vi "WT500 Read Power.vi"(0 "VISA resource name":refnum<visa-resource-name>="WT500", 1 "WT500 CMDS":T1, 5 "V Range (8: 1000V)":u16(ring)=6 items=["AUTO", "15", "30", "60", "100", "150", "300", "600", "1000", "7.5", "15", "30", "50", "75", "150", "300", "500"], 7 "I Range (7: 40A)":u16(ring)=7 items=["AUTO", "500 mA", "1 A", "2 A", "5 A", "10 A", "20 A", "40 A", "S-AUTO", "50 mV", "100 mV", "200 mV", "500 mV", "1 V", "2 V", "5 V", "10 V", "250 mA", "500 mA", "1 A", "2.5 A", "5 A", "10 A", "20 A", "25 mV", "50 mV", "100 mV", "250 mV", "500 mV", "1 V", "2.5 V", "5 V"], 11 "error in (no error)":errorcluster) -> (4 "VISA resource name out":refnum<visa-resource-name>="WT500", 6 "PowerData":T2={"Current L1"=236.2, "Current L2"=17.749, "Power"=4192.0, "WattHours"=0.0, "Voltage L2"=236.2, "Voltage L1"=236.2}, 8 "Error Message":string, 10 "Measurement Values":dbl[](array[numeric]) format="%.4p", 14 "Label":string[](array[string])=["Urms:Element 1", "Urms:Element 2", "Irms:Element 1", "Irms:Element 2", "P:Sigma", "Wp:Sigma", "I +peak:Element 1", "I +peak:Element 2"], 15 "error out":errorcluster)   [LabVIEW 2012]
uses:
  Dryer PowerData.ctl
  WT500 Sequences.ctl
  Drivers/Yokogawa WT200 Series/Yokogawa WT200 Series.lvlib
panel:
  out "Error Message 2":string
  out "(Max Current)":dbl
  in  "Pole":u16(ring)=1 items=["NONE", "Element 1", "Element 2", "Element 3", "Sigma"]
  in  "Measurement":u16(ring)=1 items=["None", "Urms", "Umn", "Udc", "Urmn", "Uac", "Irms", "Imn", "Idc", "Irmn", "Iac", "P", "S", "Q", "Lambda", "Phi", "Freq U", "Freq I", "U +peak", "U -peak", "I +peak", "I -peak", "Cf U", "Cf I", "Time", "Wp", "Wp+", "Wp-", "q", "q+", "q-", "WS", "WQ", "Eta 1", "Eta 2", "F1", "F2", "F3", "F4", "F5", "F6", "F7", "F8", "U(k)", "I(k)", "P(k)", "S(k)", "Q(k)", "Lambda(k)", "Phi(k)", "Phi U(k)", "Phi I(k)", "Uhdf(k)", "Ihdf(k)", "Phdf(k)", "Uthd", "Ithd", "Pthd", "Phi Ui-Uj", "Phi Ui-Uk", "Phi Ui-Ii", "Phi Ui-Ij", "Phi Ui-Ik", "Delta 1", "Delta 2", "Delta 3", "Delta 4"]
  out "Data Length":i32
  out "Read Data":string
  in  "Write Data":string
  out "Scan Error":bool
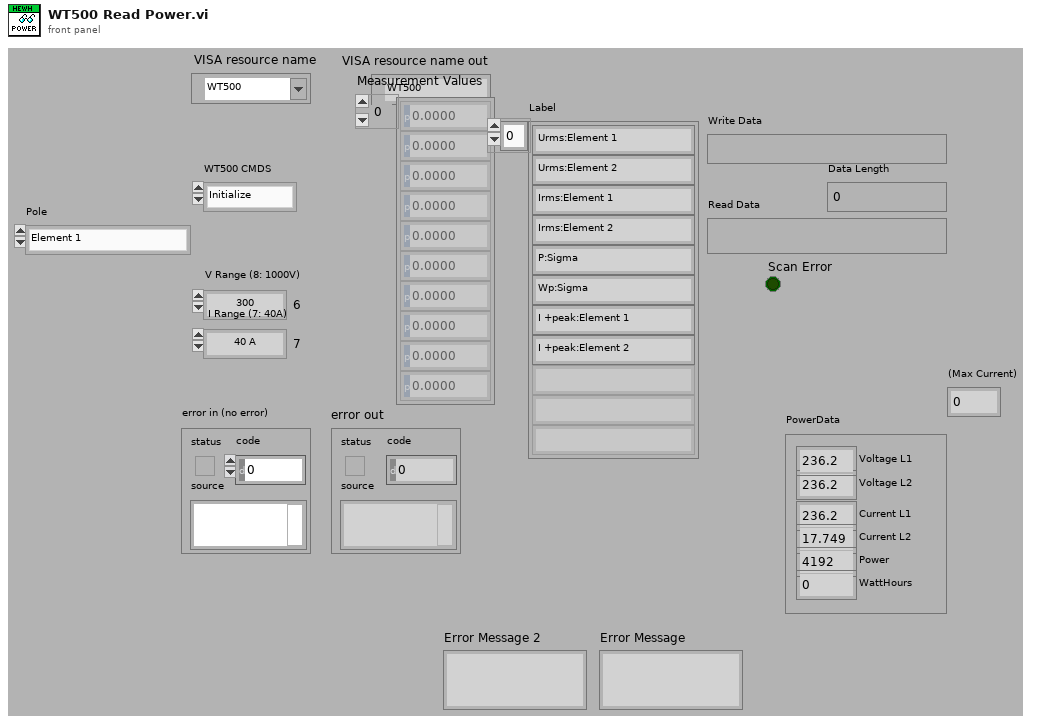
[diagram p1: front panel]
types:
  T1 = typedef "WT500 Sequences.ctl" = enum16{"Initialize", "GetReadings", "GetErrors", "Close", "NoOp", "MiscCmd"}
  T2 = typedef "Dryer PowerData.ctl" = cluster{"Current L1":dbl, "Current L2":dbl, "Power":dbl, "WattHours":dbl, "Voltage L2":dbl, "Voltage L1":dbl}
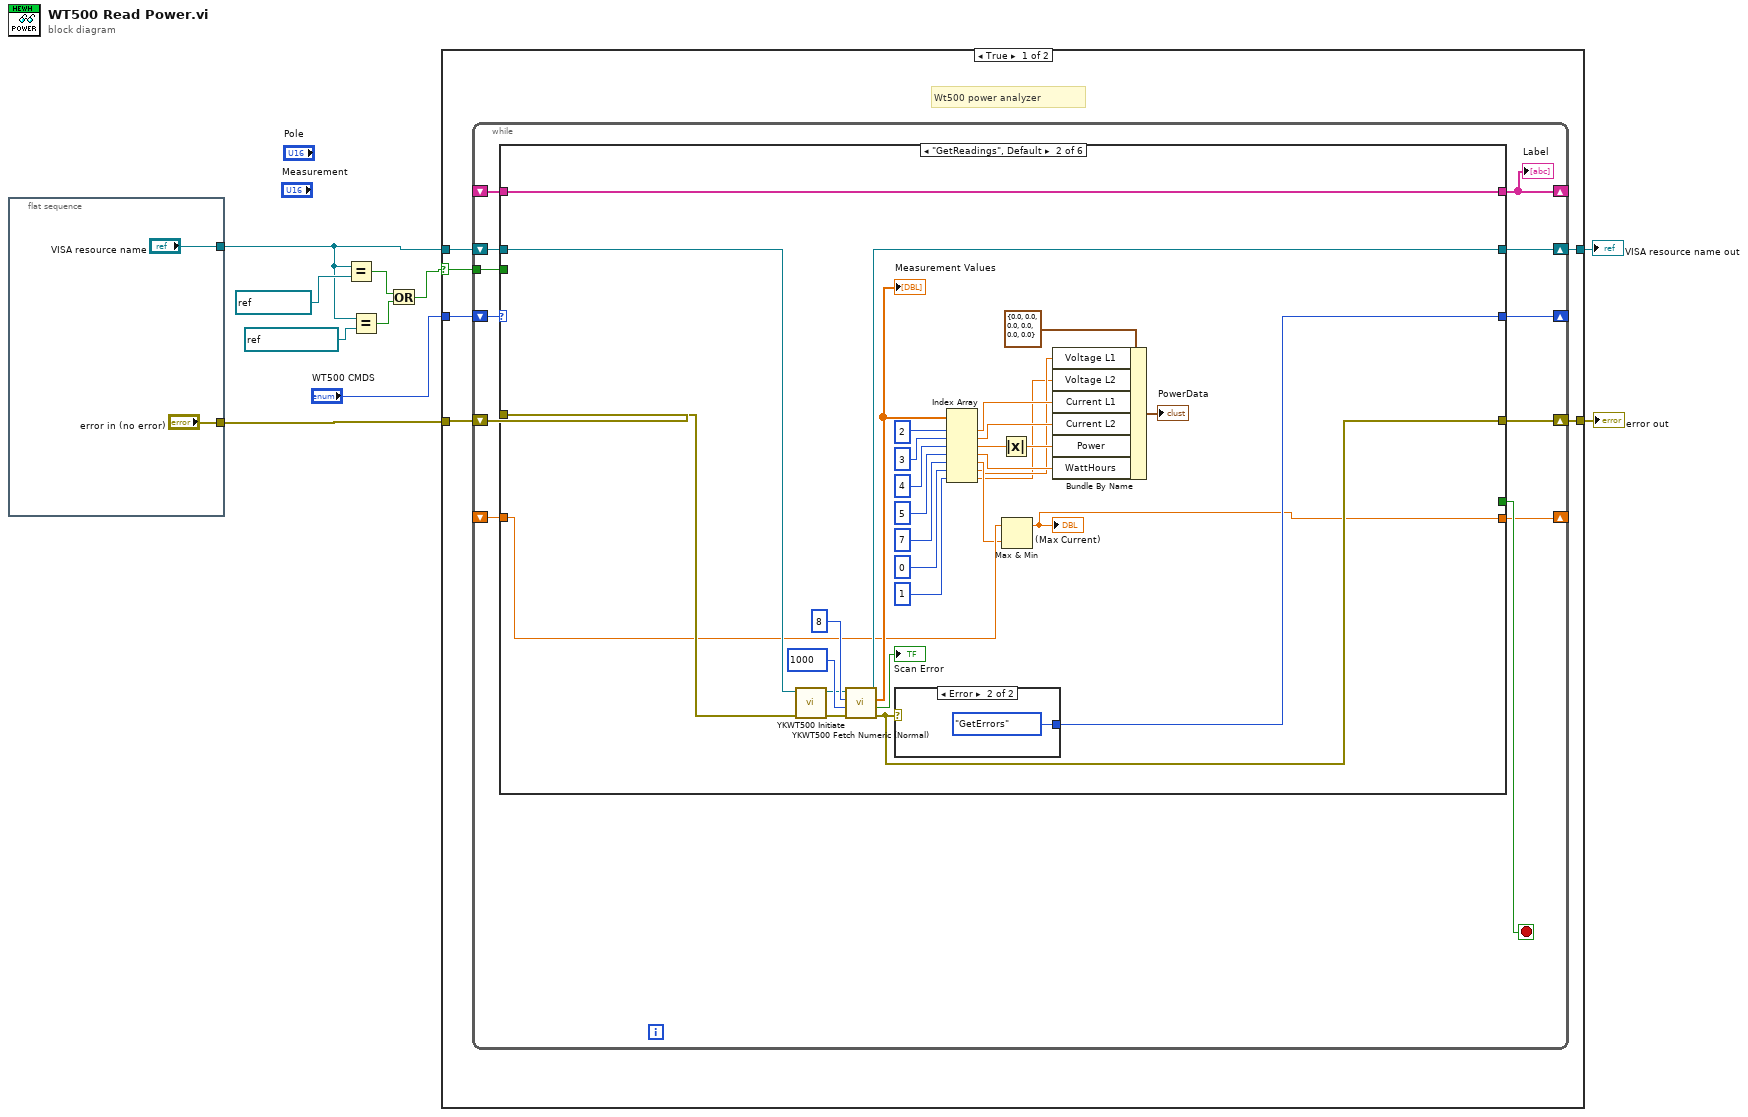
[diagram p0: block diagram]
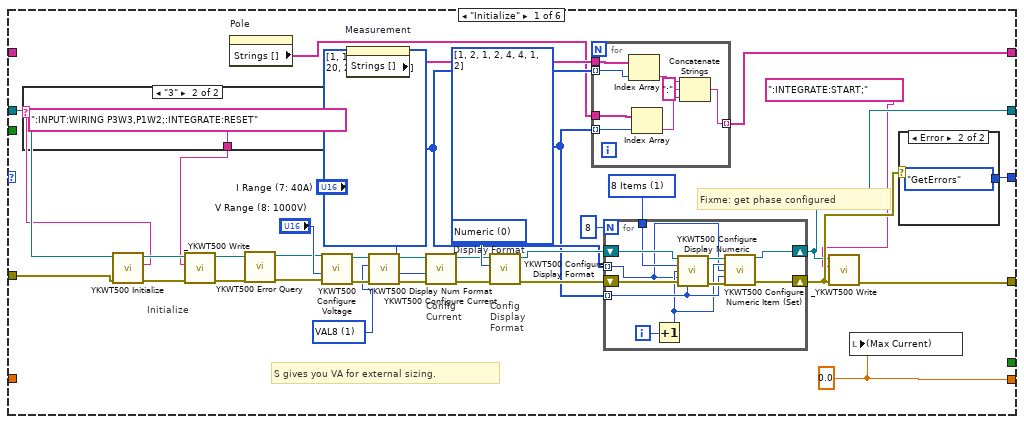
[diagram p2: hidden frame]
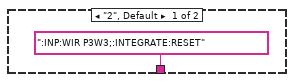
[diagram p3: hidden frame]
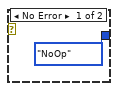
[diagram p4: hidden frame]
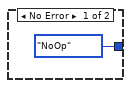
[diagram p5: hidden frame]
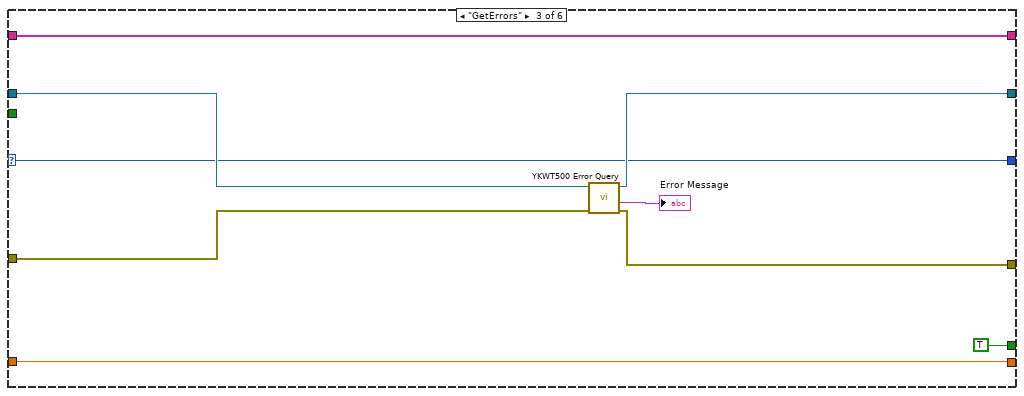
[diagram p6: hidden frame]
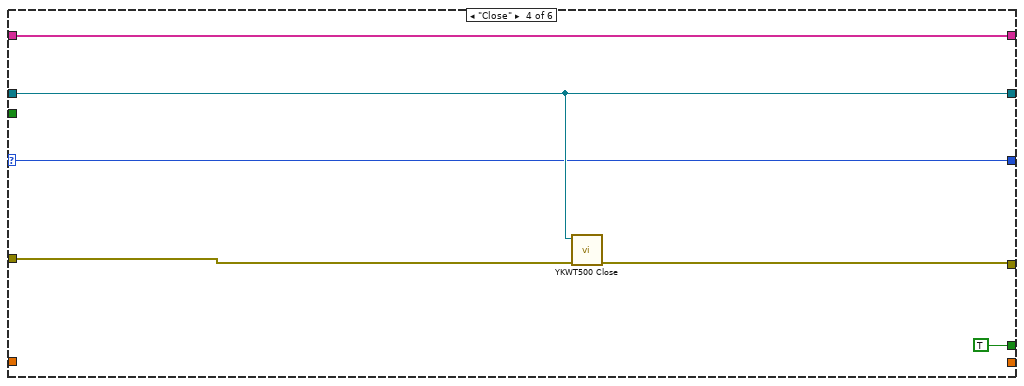
[diagram p7: hidden frame]
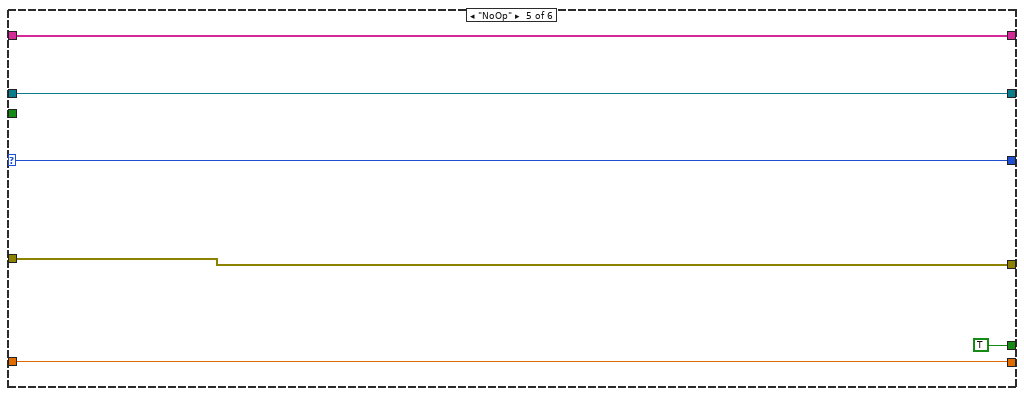
[diagram p8: hidden frame]
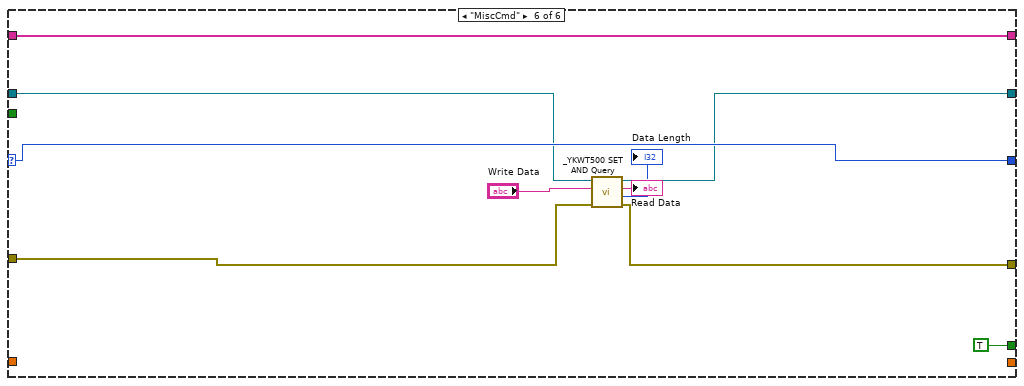
[diagram p9: hidden frame]
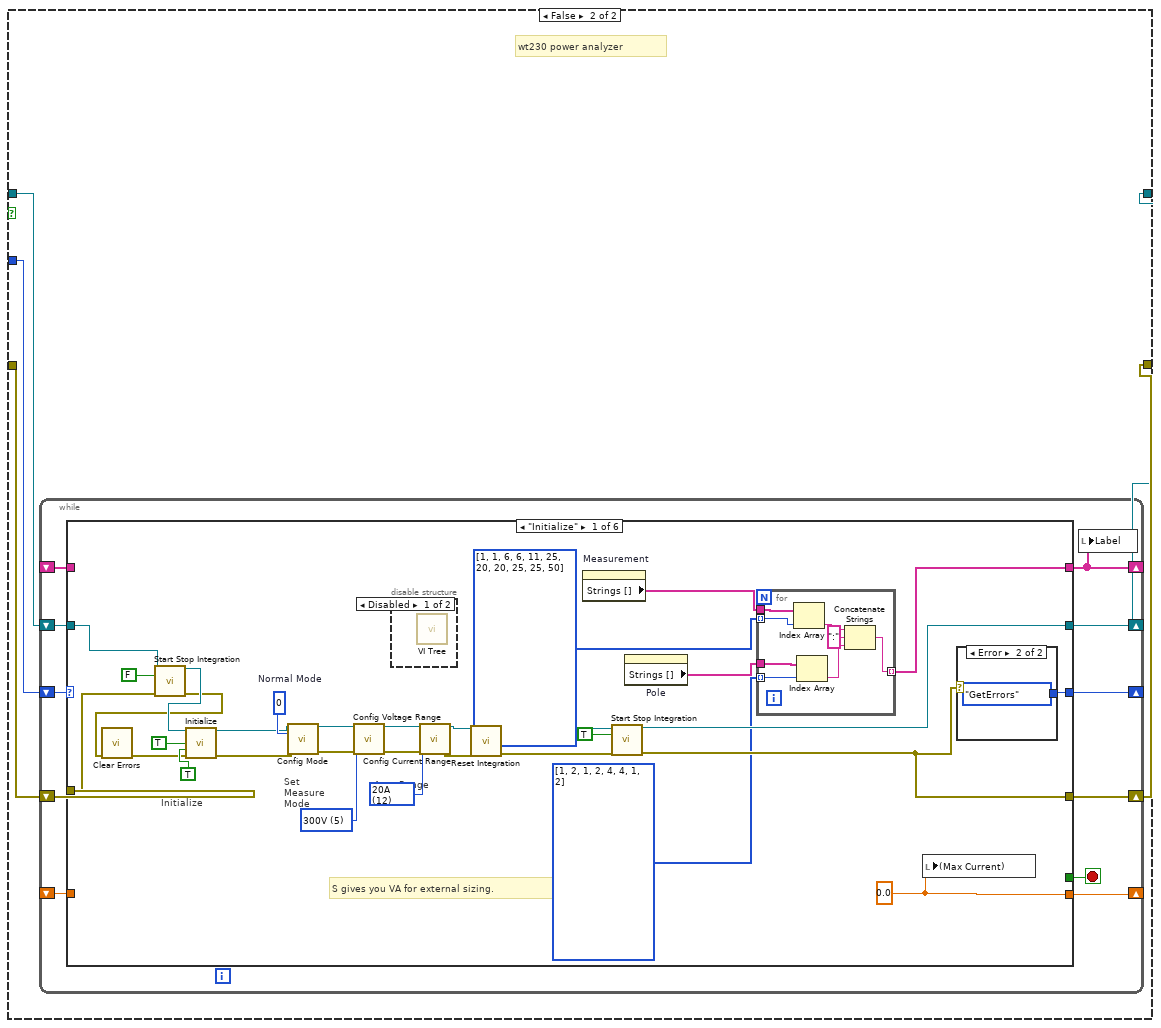
[diagram p10: hidden frame]
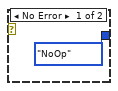
[diagram p12: hidden frame]
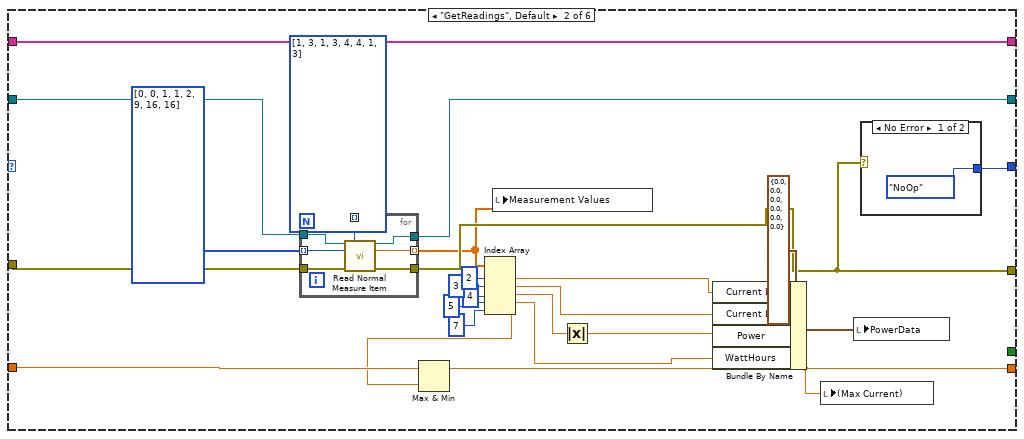
[diagram p13: hidden frame]
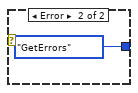
[diagram p14: hidden frame]
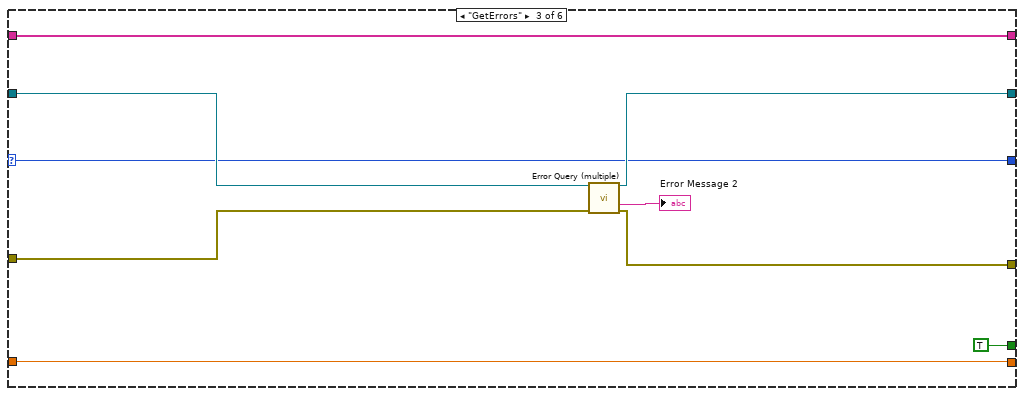
[diagram p15: hidden frame]
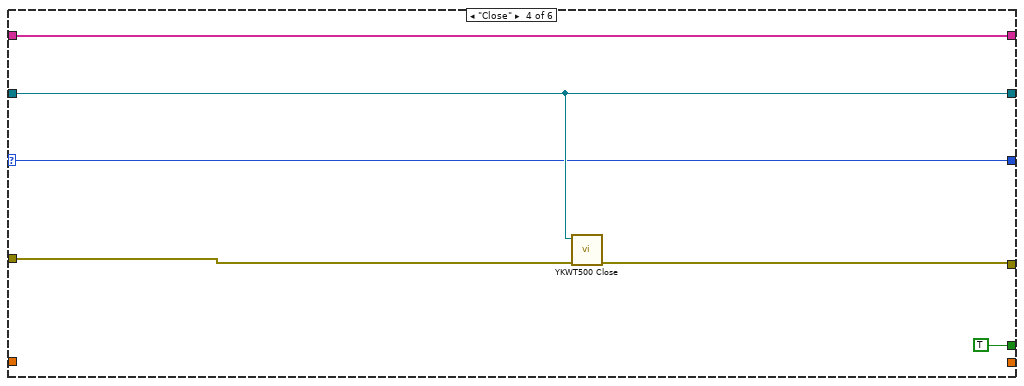
[diagram p16: hidden frame]
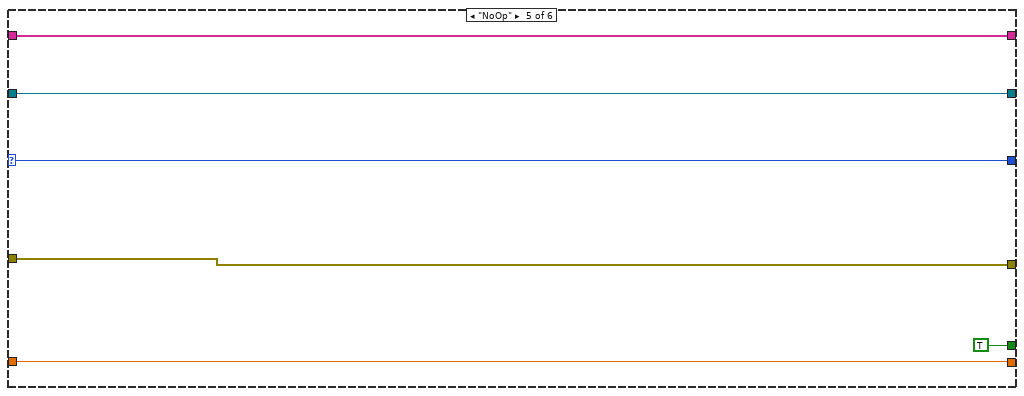
[diagram p17: hidden frame]
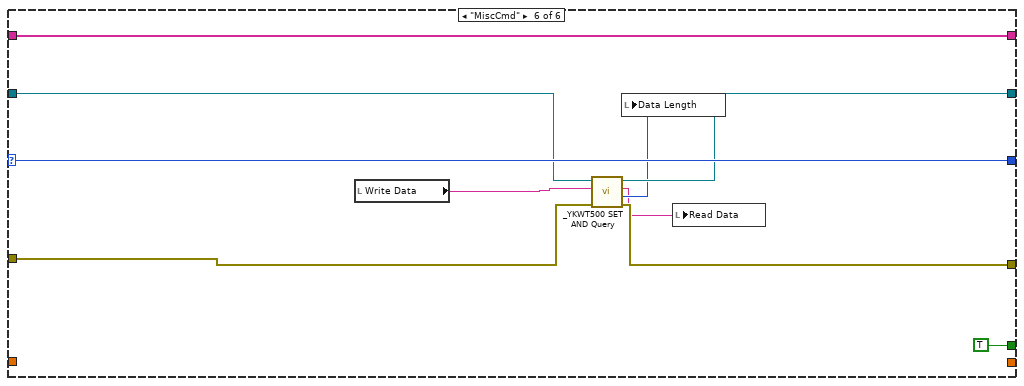
[diagram p18: hidden frame]
diagram:
  n1 = flat-sequence {
    tunnel: ["error in (no error)"] -> w7
    tunnel: ["VISA resource name"] -> w5
    frame #0 {
    }
  }
  n2 = Equal?(x=w5, y=refnum<visa-resource-name> "WT500" ("VISA resource name")) -> (x = y?=w2:bool)
  n3 = Equal?(x=w5, y=refnum<visa-resource-name> "YGWT500" ("VISA resource name")) -> (x = y?=w3:bool)
  n4 = Or(x=w2, y=w3) -> (x .or. y?=w1:bool)
  n5 = case shown="True" w1 {
    selector: w1 -> [w13 _]
    tunnel: "WT500 CMDS" -> [w18 w157]
    tunnel: w7 -> [w17 w156]
    tunnel: [w16 w155] -> w9
    tunnel: w5 -> [w15 w154]
    tunnel: [w14 w153] -> w8
    frame True {
      # "Wt500 power analyzer"
      n6 = while {
        shift-right: [w28] -> w16
        shift-left: w17 -> [w29]
        shift-right: [w26] -> _
        shift-left: w18 -> [w30]
        shift-right: [w24] -> w14
        shift-left: w15 -> [w25]
        shift-right: [w22] -> _
        shift-left: _ -> [w23]
        shift-right: [w21] -> _
        shift-left: _ -> [w20]
        tunnel: w13 -> [w19]
        stop <- w27 stop-if-true
        n7 = case shown="\"GetReadings\", Default" w30 {
          selector: w30 -> [_ _ w126 w133 w140 w151]
          tunnel: w29 -> [w60 w100 w128 w136 w141 w148]
          tunnel: [w37 w103 w124 w135 w141 w147] -> w28
          tunnel: [_ _ TRUE TRUE TRUE TRUE] -> w27
          tunnel: [w59 w102 w126 w133 w140 w151] -> w26
          tunnel: w25 -> [w58 w101 w130 w134 w139 w150]
          tunnel: [w38 w104 w129 w134 w139 w149] -> w24
          tunnel: [w44 w97 w123 w131 w138 w143] -> w22
          tunnel: w23 -> [_ w97 w123 w131 w138 w143]
          tunnel: [w40 w93 w122 _ w137 _] -> w21
          tunnel: w20 -> [_ w95 w122 _ w137 _]
          tunnel: w19 -> [_ _ _ _ _ _]
          frame "Initialize" {
            w40 = 0.0
            w49 = u16 1 items=["VAL4", "VAL8", "VAL16", "MATRIX", "ALL"] ("Display Format (0: Numeric)")
            w46 = u16[] [1, 2, 1, 2, 4, 4, 1, 2] items=["NONE", "Element 1", "Element 2", "Element 3", "Sigma"]
            w48 = u16[] [1, 1, 6, 6, 11, 25, 20, 20, 25, 25, 50] items=["None", "Urms", "Umn", "Udc", "Urmn", "Uac", "Irms", "Imn", "Idc", "Irmn", "Iac", "P", "S", "Q", "Lambda", "Phi", "Freq U", "Freq I", "U +peak", "U -peak", "I +peak", "I -peak", "Cf U", "Cf I", "Time", "Wp", "Wp+", "Wp-", "q", "q+", "q-", "WS", "WQ", "Eta 1", "Eta 2", "F1", "F2", "F3", "F4", "F5", "F6", "F7", "F8", "U(k)", "I(k)", "P(k)", "S(k)", "Q(k)", "Lambda(k)", "Phi(k)", "Phi U(k)", "Phi I(k)", "Uhdf(k)", "Ihdf(k)", "Phdf(k)", "Uthd", "Ithd", "Pthd", "Phi Ui-Uj", "Phi Ui-Uk", "Phi Ui-Ii", "Phi Ui-Ij", "Phi Ui-Ik", "Delta 1", "Delta 2", "Delta 3", "Delta 4"] ("Array of Measurements")
            w55 = u16 1 items=["4 Items", "8 Items", "16 Items", "Matrix"] ("Numeric Format (0: 4 Items)")
            w65 = u16 0 items=["Numeric", "Wave", "Bar", "Vector", "Trend"]  # Display Format
            # "S gives you VA for external sizing."
            # "Fixme: get phase configured"
            # "Config\nDisplay\nFormat"
            # "Config\nCurrent"
            # "Config\nVoltage"
            # "Initialize"
            n8 = call "YKWT500 Initialize.vi"("error in (no error)"=w60, "VISA resource name"=w58) -> ("error out"=w42:errorcluster, "Num Cards"=w31:string, "VISA resource name out"=w43:refnum<visa-resource-name>)  [unwired: 7 in]
            n9 = case shown="\"3\"" w31 {
              tunnel: [":INP:WIR P3W3;:INTEGRATE:RESET" ("Write Data") ":INPUT:WIRING P3W3,P1W2;:INTEGRATE:RESET" ("Write Data")] -> w41
              frame "2", Default {
              }
              frame "3" {
              }
            }
            n10 = call "_YKWT500 Write.vi"("error in (no error)"=w42, "Write Data"=w41, "VISA resource name"=w43) -> ("error out"=w35:errorcluster, "VISA resource name out"=w34:refnum<visa-resource-name>)  [unwired: 5 in, 2 out]
            n11 = property on="Pole" class="Ring (strict)"() -> ("Strings []"=w45:string[])  [unwired: 2 in, 2 out]
            n12 = call "YKWT500 Error Query.vi"("error in (no error)"=w35, "VISA resource name"=w34) -> ("error out"=w32:errorcluster, "VISA resource name out"=w33:refnum<visa-resource-name>)  [unwired: 6 in, 2 out]
            n13 = call "YKWT500 Configure Voltage.vi"("error in (no error)"=w32, "Voltage Range (8: 1000V)"="V Range (8: 1000V)", "VISA resource name"=w33) -> ("error out"=w53:errorcluster, "VISA resource name out"=w50:refnum<visa-resource-name>)  [unwired: 7 in]
            n14 = property on="Measurement" class="Ring (strict)"() -> ("Strings []"=w47:string[])  [unwired: 2 in, 2 out]
            n15 = call "YKWT500 Display Num Format.vi"("error in (no error)"=w53, "Display Format (0: Numeric)"=w49, "VISA resource name"=w50) -> ("error out"=w52:errorcluster, "VISA resource name out"=w51:refnum<visa-resource-name>)  [unwired: 7 in]
            n16 = call "YKWT500 Configure Current.vi"("error in (no error)"=w52, "Current Range (7: 40A)"="I Range (7: 40A)", "VISA resource name"=w51) -> ("error out"=w64:errorcluster, "VISA resource name out"=w63:refnum<visa-resource-name>)  [unwired: 7 in]
            n17 = call "YKWT500 Configure Display Format.vi"("error in (no error)"=w64, "Display Format (0: Numeric)"=w65, "VISA resource name"=w63) -> ("error out"=w56:errorcluster, "VISA resource name out"=w57:refnum<visa-resource-name>)  [unwired: 7 in]
            n18 = for {
              tunnel: w48 -> [w75] mode=indexing
              tunnel: w47 -> [w74]
              tunnel: w46 -> [w73] mode=indexing
              tunnel: w45 -> [w72]
              tunnel: [w68] -> w44 mode=indexing
              n19 = Index Array(array=w74, index=w75) -> (element=w71:string)
              n20 = Index Array(array=w72, index=w73) -> (element=w69:string)
              n21 = Concatenate Strings(w71, ":" ("string"), w69) -> (w68:string)
            }
            n22 = for {
              N: 8 -> [_]
              shift-right: [w80] -> w38
              shift-left: w57 -> [w86]
              shift-right: [w81] -> w39
              shift-left: w56 -> [w85]
              tunnel: w55 -> [w83]
              tunnel: w46 -> [w78] mode=indexing
              tunnel: w48 -> [w76] mode=indexing
              i -> [w84]
              n23 = Increment(x=w84) -> (x+1=w77:i32)
              n24 = call "YKWT500 Configure Display Numeric.vi"("VISA resource name"=w86, "Numeric Format (0: 4 Items)"=w83, "Numeric Item Number (1)"=w77, "Numeric Function (0: None)"=w76, "error in (no error)"=w85, "Element (1: Element 1)"=w78) -> ("VISA resource name out"=w79:refnum<visa-resource-name>, "error out"=w82:errorcluster)  [unwired: 8 in]
              n25 = call "YKWT500 Configure Numeric Item (Set).vi"("VISA resource name"=w79, "Numeric Item Number (1)"=w77, "Numeric Function (0: None)"=w76, "Element (1: Element 1)"=w78, "error in (no error)"=w82) -> ("VISA resource name out"=w80:refnum<visa-resource-name>, "error out"=w81:errorcluster)  [unwired: 9 in]
            }
            n26 = call "_YKWT500 Write.vi"("error in (no error)"=w39, "Write Data"=":INTEGRATE:START;", "VISA resource name"=w38) -> ("error out"=w37:errorcluster)  [unwired: 5 in, 3 out]
            n27 = local write "(Max Current)"(w40) -> ()
            n28 = case shown="Error" w39 {
              tunnel: [WT500_Sequences."NoOp" ("WT500 CMDS") WT500_Sequences."GetErrors" ("WT500 CMDS")] -> w59
              frame No Error {
              }
              frame Error {
              }
            }
          }
          frame "GetReadings", Default {
            n29 = call "YKWT500 Initiate.vi"("error in (no error)"=w100, "VISA resource name"=w101) -> ("error out"=w98:errorcluster, "VISA resource name out"=w99:refnum<visa-resource-name>)  [unwired: 8 in]
            n30 = call "YKWT500 Fetch Numeric (Normal).vi"("error in (no error)"=w98, "Timeout (10000 ms)"=u32 1000, "Number of Item (255)"=8, "VISA resource name"=w99) -> ("error out"=w103:errorcluster, "Scan Error"=→"Scan Error":bool, "Measurement Value"=w108:dbl[], "VISA resource name out"=w104:refnum<visa-resource-name>)  [unwired: 4 in]
            "Measurement Values" <- w108
            n31 = case shown="Error" w103 {
              tunnel: [WT500_Sequences."NoOp" ("WT500 CMDS") WT500_Sequences."GetErrors" ("WT500 CMDS")] -> w102
              frame No Error {
              }
              frame Error {
              }
            }
            n32 = Index Array(array=w108, index #1=2 ("index"), index #2=3 ("index"), index #3=4 ("index"), index #4=5 ("index"), index #5=7 ("index"), index #6=0 ("index"), index #7=1 ("index")) -> (element #1=w118:dbl, element #2=w117:dbl, element #3=w112:dbl, element #4=w115:dbl, element #5=w94:dbl, element #6=w90:dbl, element #7=w89:dbl)
            n33 = Absolute Value(x=w112) -> (abs(x)=w116:dbl)
            n34 = Max & Min(x=w95, y=w94) -> (max(x,y)=w93:dbl)  [unwired: 1 out]
            "(Max Current)" <- w93
            n35 = Bundle By Name(cluster=T2 {"Current L1"=0.0, "Current L2"=0.0, "Power"=0.0, "WattHours"=0.0, "Voltage L2"=0.0, "Voltage L1"=0.0} ("PowerData"), "Voltage L1"=w90, "Voltage L2"=w89, "Current L1"=w118, "Current L2"=w117, "Power"=w116, "WattHours"=w115) -> (→"PowerData":T2)
          }
          frame "GetErrors" {
            n36 = call "YKWT500 Error Query.vi"("error in (no error)"=w128, "VISA resource name"=w130) -> ("error out"=w124:errorcluster, "Error Message"=→"Error Message":string, "VISA resource name out"=w129:refnum<visa-resource-name>)  [unwired: 6 in, 1 out]
          }
          frame "Close" {
            n37 = call "YKWT500 Close.vi"("error in (no error)"=w136, "VISA resource name"=w134) -> ("error out"=w135:errorcluster)  [unwired: 9 in]
          }
          frame "NoOp" {
          }
          frame "MiscCmd" {
            n38 = call "_YKWT500 SET AND Query.vi"("error in (no error)"=w148, "Write Data"="Write Data", "VISA resource name"=w150) -> ("error out"=w147:errorcluster, "Data Length"=→"Data Length":i32, "Read Data"=→"Read Data":string, "VISA resource name out"=w149:refnum<visa-resource-name>)  [unwired: 5 in]
          }
        }
        "Label" <- w22
      }
    }
    frame False {
      # "wt230 power analyzer"
      n39 = while {
        shift-right: [w166] -> w155
        shift-left: w156 -> [w167]
        shift-right: [w164] -> _
        shift-left: w157 -> [w168]
        shift-right: [w162] -> w153
        shift-left: w154 -> [w163]
        shift-right: [w158] -> _
        shift-left: _ -> [w161]
        shift-right: [w160] -> _
        shift-left: _ -> [w159]
        stop <- w165 stop-if-true
        n40 = case shown="\"Initialize\"" w168 {
          selector: w168 -> [_ _ w247 w254 w261 w272]
          tunnel: w167 -> [w171 w214 w249 w257 w262 w269]
          tunnel: [w186 w213 w245 w256 w262 w268] -> w166
          tunnel: [_ _ TRUE TRUE TRUE TRUE] -> w165
          tunnel: [w199 w223 w247 w254 w261 w272] -> w164
          tunnel: w163 -> [w175 w217 w251 w255 w260 w271]
          tunnel: [w187 w212 w250 w255 w260 w270] -> w162
          tunnel: [w191 w210 w244 w252 w259 w267] -> w158
          tunnel: w161 -> [_ w210 w244 w252 w259 w267]
          tunnel: [w192 w218 w243 _ w258 _] -> w160
          tunnel: w159 -> [_ w221 w243 _ w258 _]
          frame "Initialize" {
            w183 = u16 12 items=["Auto", "5mA", "10mA", "20mA", "50mA", "100mA", "200mA", "0.5A", "1A", "2A", "5A", "10A", "20A", "50mV", "100mV", "200mV", "2.5V", "5V", "10V"] ("A Range (12: 20A)")
            w184 = u16 5 items=["Auto", "15V", "30V", "60V", "150V", "300V", "600V"] ("V Range (6: 600V)")
            w177 = u16[] [1, 2, 1, 2, 4, 4, 1, 2] items=["NONE", "Element 1", "Element 2", "Element 3", "Sigma"]
            w178 = u16[] [1, 1, 6, 6, 11, 25, 20, 20, 25, 25, 50] items=["None", "Urms", "Umn", "Udc", "Urmn", "Uac", "Irms", "Imn", "Idc", "Irmn", "Iac", "P", "S", "Q", "Lambda", "Phi", "Freq U", "Freq I", "U +peak", "U -peak", "I +peak", "I -peak", "Cf U", "Cf I", "Time", "Wp", "Wp+", "Wp-", "q", "q+", "q-", "WS", "WQ", "Eta 1", "Eta 2", "F1", "F2", "F3", "F4", "F5", "F6", "F7", "F8", "U(k)", "I(k)", "P(k)", "S(k)", "Q(k)", "Lambda(k)", "Phi(k)", "Phi U(k)", "Phi I(k)", "Uhdf(k)", "Ihdf(k)", "Phdf(k)", "Uthd", "Ithd", "Pthd", "Phi Ui-Uj", "Phi Ui-Uk", "Phi Ui-Ii", "Phi Ui-Ij", "Phi Ui-Ik", "Delta 1", "Delta 2", "Delta 3", "Delta 4"] ("Array of Measurements")
            w193 = u16 0  # Normal Mode
            w192 = 0.0
            # "Initialize"
            # "Auto Range"
            # "Set \nMeasure \nMode"
            # "S gives you VA for external sizing."
            n41 = call "Start Stop Integration.vi"("VISA resource name"=w175, "Start/Stop (F: Stop)"=FALSE, "error in (no error)"=w171) -> ("VISA resource name out"=w174:refnum<visa-resource-name>, "error out"=w170:errorcluster)  [unwired: 11 in]
            n42 = call <vilib>:"Clear Errors.vi"("error in (no error)"=w170) -> ("error out"=w169:errorcluster)  [unwired: 6 in]
            n43 = call "Initialize.vi"("VISA resource name"=w174, "ID Query (T: Check)"=TRUE, "Reset (T: Reset)"=TRUE, "error in (no error)"=w169) -> ("VISA resource name out"=w173:refnum<visa-resource-name>, "error out"=w172:errorcluster)  [unwired: 10 in]
            n44 = call "Config Mode.vi"("VISA resource name"=w173, "Mode (0: RMS)"=w193, "error in (no error)"=w172) -> ("VISA resource name out"=w196:refnum<visa-resource-name>, "error out"=w197:errorcluster)  [unwired: 11 in]
            n45 = call "Config Voltage Range.vi"("VISA resource name"=w196, "V Range (6: 600V)"=w184, "error in (no error)"=w197) -> ("VISA resource name out"=w195:refnum<visa-resource-name>, "error out"=w194:errorcluster)  [unwired: 11 in]
            n46 = disable-structure shown="Disabled" {
              frame Disabled {
                n47 = call <instrlib>:"VI Tree.vi"() -> ()  [unwired: 12 in]
              }
              frame Enabled {
              }
            }
            n48 = call "Config Current Range.vi"("VISA resource name"=w195, "A Range (12: 20A)"=w183, "error in (no error)"=w194) -> ("VISA resource name out"=w182:refnum<visa-resource-name>, "error out"=w190:errorcluster)  [unwired: 11 in]
            n49 = call "Reset Integration.vi"("VISA resource name"=w182, "error in (no error)"=w190) -> ("VISA resource name out"=w188:refnum<visa-resource-name>, "error out"=w189:errorcluster)  [unwired: 12 in]
            n50 = property on="Measurement" class="Ring (strict)"() -> ("Strings []"=w181:string[])  [unwired: 2 in, 2 out]
            n51 = call "Start Stop Integration.vi"("VISA resource name"=w188, "Start/Stop (F: Stop)"=TRUE, "error in (no error)"=w189) -> ("VISA resource name out"=w187:refnum<visa-resource-name>, "error out"=w186:errorcluster)  [unwired: 11 in]
            n52 = property on="Pole" class="Ring (strict)"() -> ("Strings []"=w180:string[])  [unwired: 2 in, 2 out]
            n53 = for {
              tunnel: w178 -> [w207] mode=indexing
              tunnel: w181 -> [w206]
              tunnel: w177 -> [w205] mode=indexing
              tunnel: w180 -> [w204]
              tunnel: [w200] -> w191 mode=indexing
              n54 = Index Array(array=w206, index=w207) -> (element=w203:string)
              n55 = Index Array(array=w204, index=w205) -> (element=w201:string)
              n56 = Concatenate Strings(w203, ":" ("string"), w201) -> (w200:string)
            }
            n57 = local write "(Max Current)"(w192) -> ()
            n58 = case shown="Error" w186 {
              tunnel: [WT500_Sequences."NoOp" ("WT500 CMDS") WT500_Sequences."GetErrors" ("WT500 CMDS")] -> w199
              frame No Error {
              }
              frame Error {
              }
            }
          }
          frame "GetReadings", Default {
            w216 = u16[] [1, 3, 1, 3, 4, 4, 1, 3] items=["", "Element1", "Element2", "Element3", "Sigma"]
            w215 = u16[] [0, 0, 1, 1, 2, 9, 16, 16] items=["V", "A", "W", "VA", "var", "PF", "deg", "V Hz", "A Hz", "Wh", "Wh+", "Wh-", "Ah", "Ah+", "Ah-", "Vpk", "Apk", "Math"]
            n59 = for {
              tunnel: w217 -> [w240]
              tunnel: w216 -> [w239] mode=indexing
              tunnel: w215 -> [w238] mode=indexing
              tunnel: w214 -> [w237]
              tunnel: [w236] -> w213
              tunnel: [w235] -> w212
              tunnel: [w234] -> w211 mode=indexing
              n60 = call "Read Normal Measure Item.vi"("VISA resource name"=w240, "Element (1: Element 1)"=w239, "Measure Item (0: V)"=w238, "error in (no error)"=w237) -> ("VISA resource name out"=w235:refnum<visa-resource-name>, "Measure Value"=w234:sgl, "error out"=w236:errorcluster)  [unwired: 9 in]
            }
            n61 = Index Array(array=w211, index #1=2 ("index"), index #2=3 ("index"), index #3=4 ("index"), index #4=5 ("index"), index #5=7 ("index")) -> (element #1=w232:sgl, element #2=w231:sgl, element #3=w227:sgl, element #4=w229:sgl, element #5=w220:sgl)
            n62 = Max & Min(x=w221, y=w220) -> (max(x,y)=w218:dbl)  [unwired: 1 out]
            n63 = local write "Measurement Values"(w211) -> ()
            n64 = Absolute Value(x=w227) -> (abs(x)=w230:sgl)
            n65 = Bundle By Name(cluster=T2 {"Current L1"=0.0, "Current L2"=0.0, "Power"=0.0, "WattHours"=0.0, "Voltage L2"=0.0, "Voltage L1"=0.0} ("PowerData"), "Current L1"=w232, "Current L2"=w231, "Power"=w230, "WattHours"=w229) -> (w219:T2)
            n66 = local write "(Max Current)"(w218) -> ()
            n67 = local write "PowerData"(w219) -> ()
            n68 = case shown="No Error" w213 {
              tunnel: [WT500_Sequences."NoOp" ("WT500 CMDS") WT500_Sequences."GetErrors" ("WT500 CMDS")] -> w223
              frame No Error {
              }
              frame Error {
              }
            }
          }
          frame "GetErrors" {
            n69 = call "Error Query (multiple).vi"("VISA resource name"=w251, "error in (no error)"=w249) -> ("VISA resource name out"=w250:refnum<visa-resource-name>, "Error Message"=→"Error Message 2":string, "error out"=w245:errorcluster)  [unwired: 10 in, 1 out]
          }
          frame "Close" {
            n70 = call "YKWT500 Close.vi"("error in (no error)"=w257, "VISA resource name"=w255) -> ("error out"=w256:errorcluster)  [unwired: 9 in]
          }
          frame "NoOp" {
          }
          frame "MiscCmd" {
            n71 = local read "Write Data"() -> (w266:string)
            n72 = call "_YKWT500 SET AND Query.vi"("error in (no error)"=w269, "Write Data"=w266, "VISA resource name"=w271) -> ("error out"=w268:errorcluster, "Data Length"=w265:i32, "Read Data"=w264:string, "VISA resource name out"=w270:refnum<visa-resource-name>)  [unwired: 5 in]
            n73 = local write "Data Length"(w265) -> ()
            n74 = local write "Read Data"(w264) -> ()
          }
        }
        n75 = local write "Label"(w158) -> ()
      }
    }
  }
  "error out" <- w9
  "VISA resource name out" <- w8
